vi "Is An Event Frame.vi"(7 "Event Structure index":i32, 10 "index of element":i32, 11 "Num Event Frames":i32) -> (2 "Structure Type":T1, 3 "Event Frame?":bool)   [LabVIEW 2020]
uses:
  StructureTypes.ctl
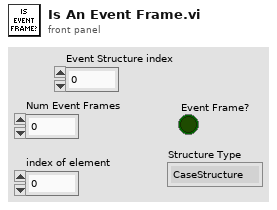
[diagram p1: front panel]
types:
  T1 = typedef "StructureTypes.ctl" = enum16{"CaseStructure", "EventStructure"}
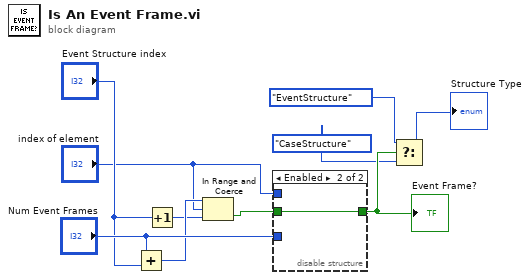
[diagram p0: block diagram]
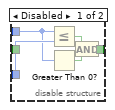
[diagram p2: hidden frame]
diagram:
  n1 = Add(x="Num Event Frames", y="Event Structure index") -> (x+y=w4:i32)
  n2 = Increment(x="Event Structure index") -> (x+1=w1:i32)
  n3 = In Range and Coerce(upper limit=w4, x="index of element", lower limit=w1) -> (In Range?=w2:bool)  [unwired: 1 out]
  n4 = disable-structure shown="Enabled" {
    disable-tunnel: [w13 w16] -> w10
    disable-tunnel: "Num Event Frames" -> [w12 _]
    disable-tunnel: "index of element" -> [w11 _]
    disable-tunnel: w2 -> [_ w16]
    frame Disabled {
      n5 = Less Or Equal?(x=w11, y=w12) -> (x <= y?=w15:bool)
      n6 = Greater Than 0?(x=w11) -> (x > 0?=w14:bool)
      n7 = And(x=w15, y=w14) -> (x .and. y?=w13:bool)
    }
    frame Enabled {
    }
  }
  "Event Frame?" <- w10
  n8 = Select(t=StructureTypes."EventStructure" ("Structure Type"), s=w10, f=StructureTypes."CaseStructure" ("Structure Type")) -> (s? t:f=→"Structure Type":T1)
